vi "从各位拟合圆创建ROI.vi"(7 "Annulus":T3={"Center X"=0, "Center Y"=0, "Inner Radius"=27, "Outer Radius"=107, "Start Angle"=0.0, "End Angle"=0.0} {"End Angle" min=-90.0 max=90.0 step=1.0 format="%.2f"; "Start Angle" min=-90.0 max=90.0 step=1.0 format="%.2f"; "Center X" scale=0.0..1024.0}, 11 "输入拟合圆信息":T2 {"Circle6"."Average SNR (dB)" format="%.2f"; "Circle6"."Average Strength" format="%.2f"; "Circle6"."Roundness (Real-World)" format="%.2f"; "Circle6"."Radius (Real-World)" format="%.2f"; "Circle6"."Center (Real-World)"."Y" format="%.2f"; "Circle6"."Center (Real-World)"."X" format="%.2f"; "Circle6"."Radius (Pixels)" format="%.2f"; "Circle6"."Center (Pixels)"."Y" format="%.2f"; "Circle6"."Center (Pixels)"."X" format="%.2f"; "Circle5"."Average SNR (dB)" format="%.2f"; "Circle5"."Average Strength" format="%.2f"; "Circle5"."Roundness (Real-World)" format="%.2f"; "Circle5"."Radius (Real-World)" format="%.2f"; "Circle5"."Center (Real-World)"."Y" format="%.2f"; "Circle5"."Center (Real-World)"."X" format="%.2f"; "Circle5"."Radius (Pixels)" format="%.2f"; "Circle5"."Center (Pixels)"."Y" format="%.2f"; "Circle5"."Center (Pixels)"."X" format="%.2f"; "Circle4"."Average SNR (dB)" format="%.2f"; "Circle4"."Average Strength" format="%.2f"; "Circle4"."Roundness (Real-World)" format="%.2f"; "Circle4"."Radius (Real-World)" format="%.2f"; "Circle4"."Center (Real-World)"."Y" format="%.2f"; "Circle4"."Center (Real-World)"."X" format="%.2f"; "Circle4"."Radius (Pixels)" format="%.2f"; "Circle4"."Center (Pixels)"."Y" format="%.2f"; "Circle4"."Center (Pixels)"."X" format="%.2f"; "Circle3"."Average SNR (dB)" format="%.2f"; "Circle3"."Average Strength" format="%.2f"; "Circle3"."Roundness (Real-World)" format="%.2f"; "Circle3"."Radius (Real-World)" format="%.2f"; "Circle3"."Center (Real-World)"."Y" format="%.2f"; "Circle3"."Center (Real-World)"."X" format="%.2f"; "Circle3"."Radius (Pixels)" format="%.2f"; "Circle3"."Center (Pixels)"."Y" format="%.2f"; "Circle3"."Center (Pixels)"."X" format="%.2f"; "Circle2"."Average SNR (dB)" format="%.2f"; "Circle2"."Average Strength" format="%.2f"; "Circle2"."Roundness (Real-World)" format="%.2f"; "Circle2"."Radius (Real-World)" format="%.2f"; "Circle2"."Center (Real-World)"."Y" format="%.2f"; "Circle2"."Center (Real-World)"."X" format="%.2f"; "Circle2"."Radius (Pixels)" format="%.2f"; "Circle2"."Center (Pixels)"."Y" format="%.2f"; "Circle2"."Center (Pixels)"."X" format="%.2f"; "Circle1"."Average SNR (dB)" format="%.2f"; "Circle1"."Average Strength" format="%.2f"; "Circle1"."Roundness (Real-World)" format="%.2f"; "Circle1"."Radius (Real-World)" format="%.2f"; "Circle1"."Center (Real-World)"."Y" format="%.2f"; "Circle1"."Center (Real-World)"."X" format="%.2f"; "Circle1"."Radius (Pixels)" format="%.2f"; "Circle1"."Center (Pixels)"."Y" format="%.2f"; "Circle1"."Center (Pixels)"."X" format="%.2f"}) -> (3 "ROIs":T1[](array[typedef]) {"Contours"."Type" items=["No Selection", "Point", "Line", "Rectangle", "Oval", "Polygon", "Freehand Region", "Annulus", "Unused2", "Unused3", "Broken Line", "Freehand Line", "Rotated Rectangle"]})   [LabVIEW 2015]
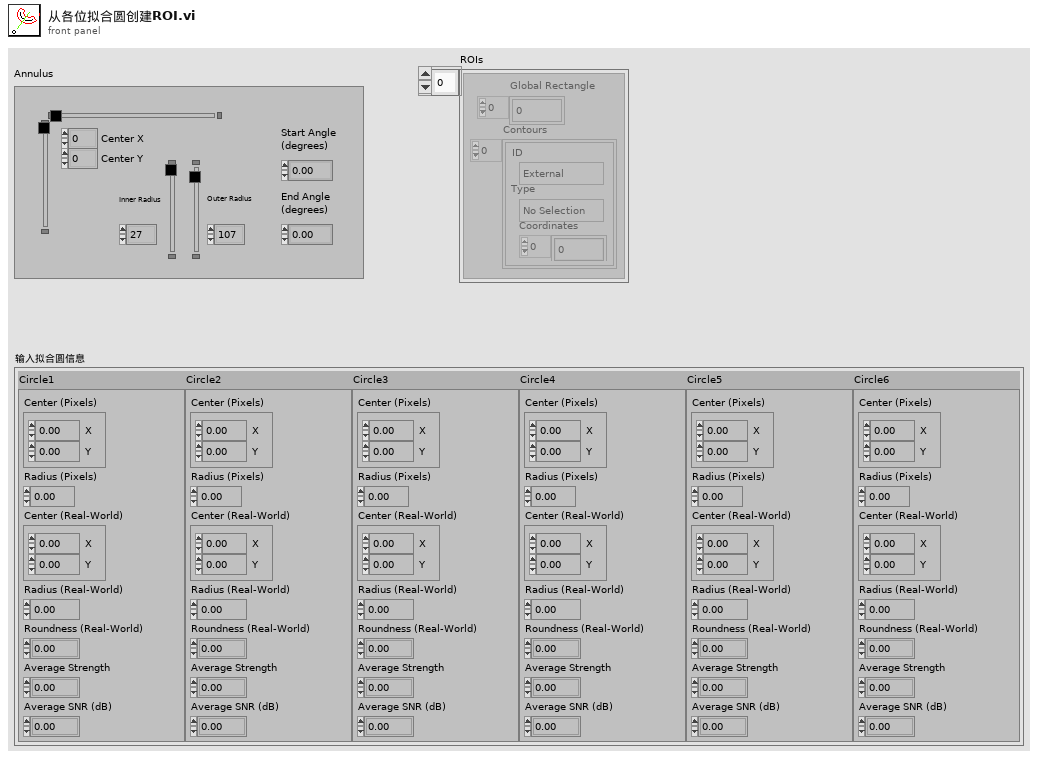
[diagram p1: front panel]
types:
  T1 = typedef "ROI Descriptor" = cluster{"Global Rectangle":i32[], "Contours":cluster{"ID":enum32{"External", "Internal"}, "Type":u32, "Coordinates":i32[]}[]}
  T2 = cluster{"Circle1":cluster{"Center (Pixels)":cluster{"X":sgl, "Y":sgl}, "Radius (Pixels)":dbl, "Center (Real-World)":cluster{"X":sgl, "Y":sgl}, "Radius (Real-World)":dbl, "Roundness (Real-World)":dbl, "Average Strength":dbl, "Average SNR (dB)":dbl}, "Circle2":cluster{"Center (Pixels)":cluster{"X":sgl, "Y":sgl}, "Radius (Pixels)":dbl, "Center (Real-World)":cluster{"X":sgl, "Y":sgl}, "Radius (Real-World)":dbl, "Roundness (Real-World)":dbl, "Average Strength":dbl, "Average SNR (dB)":dbl}, "Circle3":cluster{"Center (Pixels)":cluster{"X":sgl, "Y":sgl}, "Radius (Pixels)":dbl, "Center (Real-World)":cluster{"X":sgl, "Y":sgl}, "Radius (Real-World)":dbl, "Roundness (Real-World)":dbl, "Average Strength":dbl, "Average SNR (dB)":dbl}, "Circle4":cluster{"Center (Pixels)":cluster{"X":sgl, "Y":sgl}, "Radius (Pixels)":dbl, "Center (Real-World)":cluster{"X":sgl, "Y":sgl}, "Radius (Real-World)":dbl, "Roundness (Real-World)":dbl, "Average Strength":dbl, "Average SNR (dB)":dbl}, "Circle5":cluster{"Center (Pixels)":cluster{"X":sgl, "Y":sgl}, "Radius (Pixels)":dbl, "Center (Real-World)":cluster{"X":sgl, "Y":sgl}, "Radius (Real-World)":dbl, "Roundness (Real-World)":dbl, "Average Strength":dbl, "Average SNR (dB)":dbl}, "Circle6":cluster{"Center (Pixels)":cluster{"X":sgl, "Y":sgl}, "Radius (Pixels)":dbl, "Center (Real-World)":cluster{"X":sgl, "Y":sgl}, "Radius (Real-World)":dbl, "Roundness (Real-World)":dbl, "Average Strength":dbl, "Average SNR (dB)":dbl}}
  T3 = typedef "IMAQ Circle" = cluster{"Center X":i32, "Center Y":i32, "Inner Radius":i32, "Outer Radius":i32, "Start Angle":dbl, "End Angle":dbl}
  T4 = cluster{"Center (Pixels)":cluster{"X":sgl, "Y":sgl}, "Radius (Pixels)":dbl, "Center (Real-World)":cluster{"X":sgl, "Y":sgl}, "Radius (Real-World)":dbl, "Roundness (Real-World)":dbl, "Average Strength":dbl, "Average SNR (dB)":dbl}
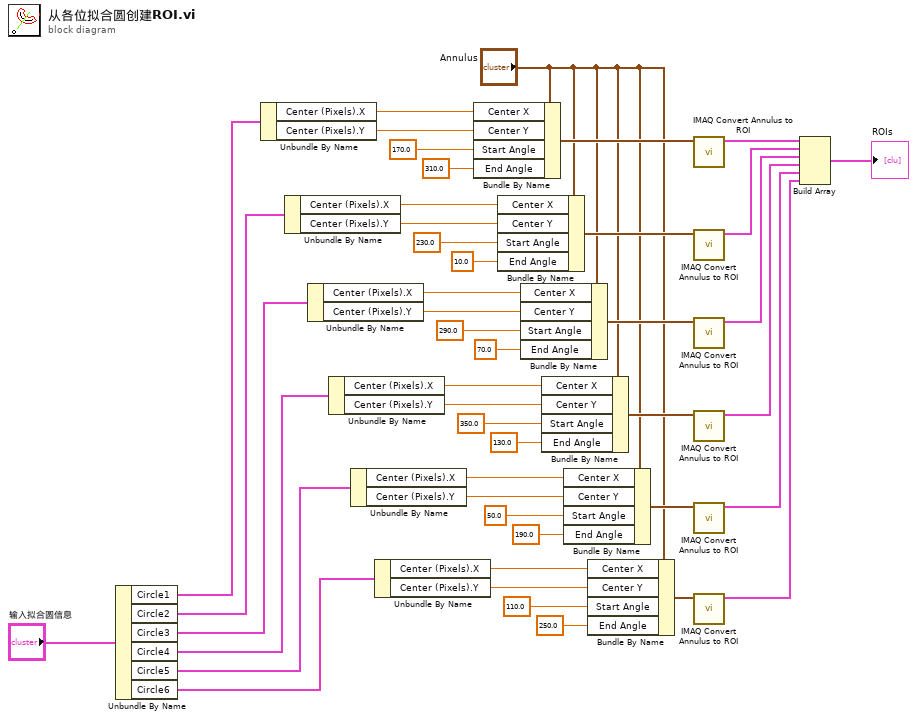
[diagram p0: block diagram]
diagram:
  n1 = Unbundle By Name("输入拟合圆信息") -> ("Circle1"=w19:T4, "Circle2"=w18:T4, "Circle3"=w17:T4, "Circle4"=w16:T4, "Circle5"=w15:T4, "Circle6"=w14:T4)
  n2 = Unbundle By Name(w19) -> ("Center (Pixels).X"=w12:sgl, "Center (Pixels).Y"=w11:sgl)
  n3 = Unbundle By Name(w18) -> ("Center (Pixels).X"=w10:sgl, "Center (Pixels).Y"=w9:sgl)
  n4 = Unbundle By Name(w17) -> ("Center (Pixels).X"=w8:sgl, "Center (Pixels).Y"=w7:sgl)
  n5 = Unbundle By Name(w16) -> ("Center (Pixels).X"=w6:sgl, "Center (Pixels).Y"=w5:sgl)
  n6 = Unbundle By Name(w15) -> ("Center (Pixels).X"=w4:sgl, "Center (Pixels).Y"=w3:sgl)
  n7 = Unbundle By Name(w14) -> ("Center (Pixels).X"=w2:sgl, "Center (Pixels).Y"=w1:sgl)
  n8 = Bundle By Name(cluster="Annulus", "Center X"=w12, "Center Y"=w11, "Start Angle"=170.0, "End Angle"=310.0) -> (w45:T3)
  n9 = Bundle By Name(cluster="Annulus", "Center X"=w10, "Center Y"=w9, "Start Angle"=230.0, "End Angle"=10.0) -> (w40:T3)
  n10 = Bundle By Name(cluster="Annulus", "Center X"=w8, "Center Y"=w7, "Start Angle"=290.0, "End Angle"=70.0) -> (w39:T3)
  n11 = Bundle By Name(cluster="Annulus", "Center X"=w6, "Center Y"=w5, "Start Angle"=350.0, "End Angle"=130.0) -> (w34:T3)
  n12 = Bundle By Name(cluster="Annulus", "Center X"=w4, "Center Y"=w3, "Start Angle"=50.0, "End Angle"=190.0) -> (w33:T3)
  n13 = Bundle By Name(cluster="Annulus", "Center X"=w2, "Center Y"=w1, "Start Angle"=110.0, "End Angle"=250.0) -> (w28:T3)
  n14 = call "IMAQ Convert Annulus to ROI"("Annulus"=w45) -> ("ROI Descriptor"=w26:T1)  [unwired: 8 in, 1 out]
  n15 = call "IMAQ Convert Annulus to ROI"("Annulus"=w40) -> ("ROI Descriptor"=w21:T1)  [unwired: 8 in, 1 out]
  n16 = call "IMAQ Convert Annulus to ROI"("Annulus"=w39) -> ("ROI Descriptor"=w22:T1)  [unwired: 8 in, 1 out]
  n17 = call "IMAQ Convert Annulus to ROI"("Annulus"=w34) -> ("ROI Descriptor"=w23:T1)  [unwired: 8 in, 1 out]
  n18 = call "IMAQ Convert Annulus to ROI"("Annulus"=w33) -> ("ROI Descriptor"=w24:T1)  [unwired: 8 in, 1 out]
  n19 = call "IMAQ Convert Annulus to ROI"("Annulus"=w28) -> ("ROI Descriptor"=w25:T1)  [unwired: 8 in, 1 out]
  n20 = Build Array(w26, w21, w22, w23, w24, w25) -> (→"ROIs":T1[])
